vi "zmq REP manual events.vi"() -> ()   [LabVIEW 2018]
uses:
  <vilib>/addons/zeromq/socket_type.ctl
  CAEN_SY527/subvis/Event Sources.ctl
  <vilib>/addons/zeromq/poll_type.ctl
  <vilib>/addons/zeromq/zmq_poll_scalar.vi
  <vilib>/addons/zeromq/zeromq.lvlib
  <vilib>/addons/zeromq/zmq_context.lvclass
  <vilib>/addons/zeromq/zmq_socket.lvclass
panel:
  in  "Send self":bool
  in  "KILL":bool
  in  "Send":bool
  out "h":bool
  out "data":string
  out "error out":errorcluster
  in  "Stop":bool
  in  "ZMQ endpoint":string="tcp://*:5555"
  # "*:5555"
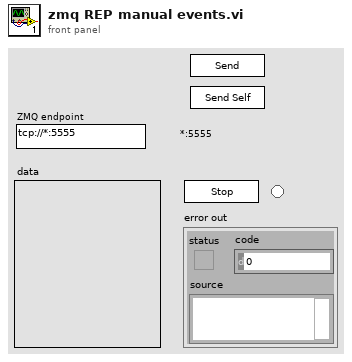
[diagram p1: front panel]
types:
  T1 = typedef "Event Sources.ctl" = enum16{"ZMQ", "INTERNAL", "Check_Errors", "Send_ZMQ_Reply", "Save_PMT_Voltages", "Set_Ramp_Voltage", "Restore PMT Voltages"}
  T2 = typedef "zeromq.lvlib/socket_type.ctl" = enum8{"ZMQ_PAIR", "ZMQ_PUB", "ZMQ_SUB", "ZMQ_REQ", "ZMQ_REP", "ZMQ_DEALER", "ZMQ_ROUTER", "ZMQ_PULL", "ZMQ_PUSH", "ZMQ_XPUB", "ZMQ_XSUB"}
  T3 = typedef "zeromq.lvlib/poll_type.ctl" = enum16{"None", "In", "Out", "In/Out"}
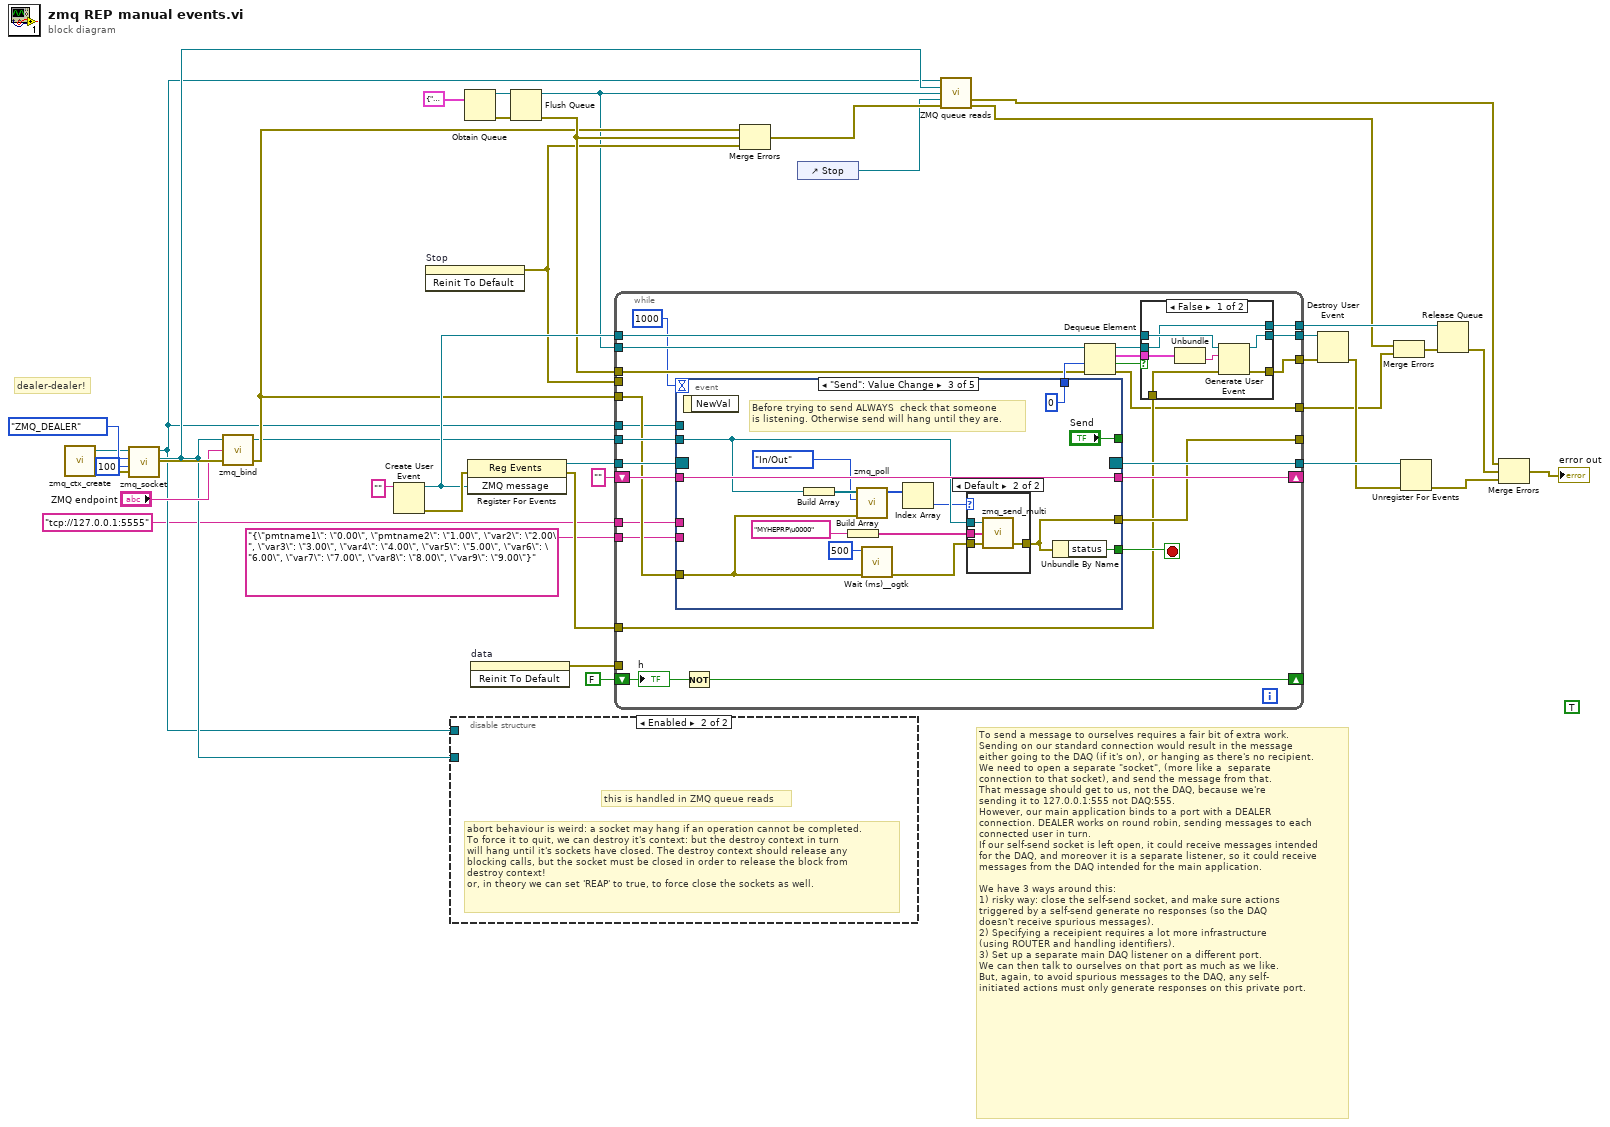
[diagram p0: block diagram]
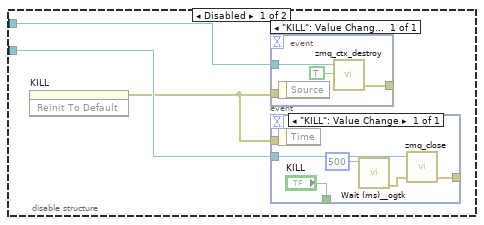
[diagram p2: hidden frame]
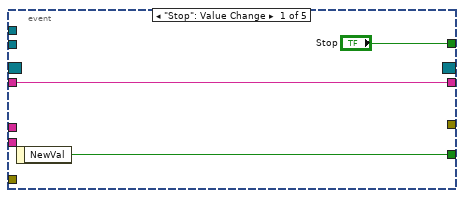
[diagram p4: hidden frame]
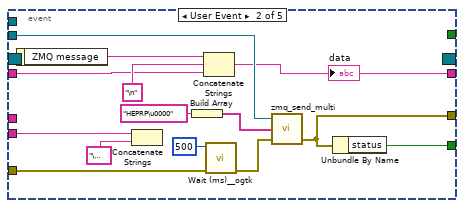
[diagram p5: hidden frame]
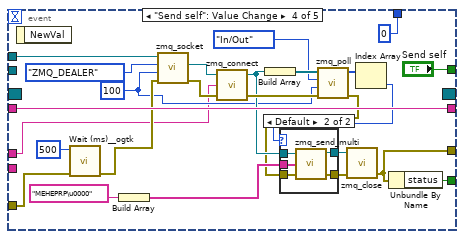
[diagram p7: hidden frame]
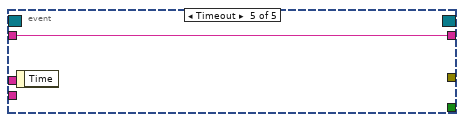
[diagram p9: hidden frame]
diagram:
  (unwired) TRUE
  # "To send a message to ourselves requires a fair bit of extra work.\nSending on our standard connection would result in the message\neither going to the DAQ (if it's on), or hanging as there's no recipient.\nWe need to open a separate \"socket\", (more like a  separate \nconnection to that socket), and send the message from that. \nThat message should get to us, not the DAQ, because we're\nsending it to 127.0.0.1:555 not DAQ:555. \nHowever, our main application binds to a port with a DEALER \nconnection. DEALER works on round robin, sending messages to each\nconnected user in turn. \nIf our self-send socket is left open, it could receive messages intended\nfor the DAQ, and moreover it is a separate listener, so it could receive \nmessages from the DAQ intended for the main application. \n\nWe have 3 ways around this:\n1) risky way: close the self-send socket, and make sure actions\ntriggered by a self-send generate no responses (so the DAQ\ndoesn't receive spurious messages). \n2) Specifying a receipient requires a lot more infrastructure \n(using ROUTER and handling identifiers). \n3) Set up a separate main DAQ listener on a different port.\nWe can then talk to ourselves on that port as much as we like.\nBut, again, to avoid spurious messages to the DAQ, any self-\ninitiated actions must only generate responses on this private port."
  # "dealer-dealer!"
  n1 = call <vilib>:"zmq_ctx_create.vi"() -> ("error out"=w40:errorcluster, "context out"=w35:refnum<class "zmq_context.lvclass">)  [unwired: 4 in]
  n2 = call <vilib>:"zmq_socket.vi"("error in"=w40, "linger (ms)"=100, "socket type"=socket_type."ZMQ_DEALER", "context in"=w35) -> ("error out"=w38:errorcluster, "socket out"=w3:refnum<class "zmq_socket.lvclass">, "context out"=w2:refnum<class "zmq_context.lvclass">)  [unwired: 1 in]
  n3 = call <vilib>:"zmq_bind.vi"("error in"=w38, "endpoint"="ZMQ endpoint", "socket in"=w3) -> ("error out"=w13:errorcluster, "socket out"=w4:refnum<class "zmq_socket.lvclass">)  [unwired: 1 in]
  n4 = Create User Event(user event datatype="" ("ZMQ message")) -> (user event=w25:refnum<user-event>, error out=w36:errorcluster)  [unwired: 1 in]
  n5 = invoke on="Stop" class="Bool (strict)" method="Reinit To Default"() -> (error out=w12:errorcluster)  [unwired: 3 in, 2 out]
  n6 = disable-structure shown="Enabled" {
    disable-tunnel: w2 -> [w43 _]
    disable-tunnel: w3 -> [w42 _]
    frame Disabled {
      n7 = invoke on="KILL" class="Bool" method="Reinit To Default"() -> (error out=w41:errorcluster)  [unwired: 3 in, 2 out]
      n8 = event shown="[0] \"KILL\": Value Change" {
        selector: _ -> [_]
        dyn-events: _ -> [_]
        timeout: _ -> [_]
        tunnel: w43 -> [w51]
        tunnel: w41 -> [_]
        tunnel: [w49] -> _
        event "KILL": Value Change {
          n9 = event-data() -> ()  [unwired: 1 in, 1 out]
          n10 = call <vilib>:"zmq_ctx_destroy.vi"("reap? (F)"=TRUE, "context in"=w51) -> ("error out"=w49:errorcluster)  [unwired: 3 in]
        }
      }
      n11 = event shown="[0] \"KILL\": Value Change" {
        selector: _ -> [_]
        dyn-events: _ -> [_]
        timeout: _ -> [_]
        tunnel: w42 -> [w48]
        tunnel: w41 -> [_]
        tunnel: ["KILL"] -> _
        tunnel: [w46] -> _
        event "KILL": Value Change {
          n12 = event-data() -> ()  [unwired: 1 in, 1 out]
          n13 = call <userlib>:"Wait (ms)__ogtk.vi"("milliseconds to wait"=u32 500) -> ("error out"=w44:errorcluster)  [unwired: 9 in, 1 out]
          n14 = call <vilib>:"zmq_close.vi"("error in"=w44, "socket"=w48) -> ("error out"=w46:errorcluster)  [unwired: 3 in]
        }
      }
    }
    frame Enabled {
      # "abort behaviour is weird: a socket may hang if an operation cannot be completed.\nTo force it to quit, we can destroy it's context: but the destroy context in turn\nwill hang until it's sockets have closed. The destroy context should release any\nblocking calls, but the socket must be closed in order to release the block from\ndestroy context! \nor, in theory we can set 'REAP' to true, to force close the sockets as well."
      # "this is handled in ZMQ queue reads"
    }
  }
  n15 = Obtain Queue(element data type=cluster{"Source":T1, "Command":string} {"Source"=enum."ZMQ", "Command"=""} ("element")) -> (queue out=w7:refnum<queue>, error out=w8:errorcluster)  [unwired: 4 in, 1 out]
  n16 = register-events(error in=w36, w25) -> (reference out=w37:refnum<event-registration>, error out=w20:errorcluster)  [unwired: 1 in]
  n17 = invoke on="data" class="Str" method="Reinit To Default"() -> (error out=w30:errorcluster)  [unwired: 3 in, 2 out]
  n18 = Flush Queue(queue=w7, error in (no error)=w8) -> (queue out=w10:refnum<queue>, error out=w14:errorcluster)  [unwired: 1 out]
  n19 = while {
    tunnel: w37 -> [w76]
    tunnel: w4 -> [w75]
    shift-right: [w73] -> _
    shift-left: "" -> [w72]
    tunnel: [w74] -> w34
    tunnel: w30 -> [_]
    shift-right: [w70] -> _
    shift-left: FALSE ("Stop") -> [w71]
    tunnel: w10 -> [w69]
    tunnel: w25 -> [w66]
    tunnel: [w65] -> w24
    tunnel: [w63] -> w23
    tunnel: [w57] -> w22
    tunnel: w20 -> [w58]
    tunnel: w14 -> [w61]
    tunnel: [w60] -> _
    tunnel: w13 -> [w59]
    tunnel: [w56] -> w16
    tunnel: w12 -> [_]
    tunnel: "{\"pmtname1\": \"0.00\", \"pmtname2\": \"1.00\", \"var2\": \"2.00\", \"var3\": \"3.00\", \"var4\": \"4.00\", \"var5\": \"5.00\", \"var6\": \"6.00\", \"var7\": \"7.00\", \"var8\": \"8.00\", \"var9\": \"9.00\"}" ("JSON string 2") -> [w54]
    tunnel: w2 -> [w53]
    tunnel: "tcp://127.0.0.1:5555" ("String") -> [w52]
    stop <- w77 stop-if-true
    n20 = event shown="[2] \"Send\": Value Change" {
      selector: w76 -> [_ _ _ _ _]
      dyn-events: [_ _ _ _ _] -> w74
      timeout: 1000 -> [_ _ _ _ _]
      tunnel: [w90 w103 w119 w149 _] -> w77
      tunnel: w75 -> [_ w104 w106 _ _]
      tunnel: [w89 w101 w112 w140 w157] -> w73
      tunnel: w72 -> [w89 w100 w112 w140 w157]
      tunnel: [_ w98 w118 w130 _] -> w60
      tunnel: [_ _ 0 ("timeout in ms (-1)") 0 ("timeout in ms (-1)") _] -> w62
      tunnel: w59 -> [_ w96 w107 w147 _]
      tunnel: w54 -> [_ w94 _ _ _]
      tunnel: ["Stop" _ "Send" "Send self" _] -> _
      tunnel: w53 -> [_ _ _ w142 _]
      tunnel: w52 -> [_ _ _ w125 _]
      event "Stop": Value Change {
        n21 = event-data() -> ("NewVal"=w90:bool)  [unwired: 1 in]
      }
      event User Event {
        n22 = event-data() -> ("ZMQ message"=w99:string)  [unwired: 1 in]
        n23 = Concatenate Strings(w94, "\u0000" ("String")) -> ()  [unwired: 1 out]
        n24 = Build Array("HEPRP\u0000" ("String")) -> (w92:string[])
        n25 = Concatenate Strings(w99, "\n" ("String"), w100) -> (w101:string)
        "data" <- w101
        n26 = call <userlib>:"Wait (ms)__ogtk.vi"("error in (no error)"=w96, "milliseconds to wait"=u32 500) -> ("error out"=w97:errorcluster)  [unwired: 8 in, 1 out]
        n27 = call <vilib>:"zmq_send_multi.vi"("error in"=w97, "parts"=w92, "socket in"=w104) -> ("error out"=w98:errorcluster)  [unwired: 1 in, 1 out]
        n28 = Unbundle By Name(w98) -> ("status"=w103:bool)
      }
      event "Send": Value Change {
        # "Before trying to send ALWAYS  check that someone\nis listening. Otherwise send will hang until they are."
        n29 = event-data() -> ()  [unwired: 1 in, 1 out]
        n30 = Build Array(w106) -> (w110:refnum<class "zmq_socket.lvclass">[])
        n31 = Build Array("MYHEPRP\u0000" ("String")) -> (w114:string[])
        n32 = call-poly <vilib>:"zmq_poll.vi"("error in"=w107, "poll type"=poll_type."In/Out", "sockets"=w110) -> ("polled events"=w109:T3[])  [unwired: 1 in, 3 out]
        n33 = call <userlib>:"Wait (ms)__ogtk.vi"("error in (no error)"=w107, "milliseconds to wait"=u32 500) -> ("error out"=w117:errorcluster)  [unwired: 8 in, 1 out]
        n34 = Index Array(array=w109) -> (element=w105:T3)  [unwired: 1 in]
        n35 = case shown="Default" w105 {
          tunnel: [w120 w124] -> w118
          tunnel: w117 -> [w120 w123]
          tunnel: w114 -> [_ w122]
          tunnel: w106 -> [_ w121]
          frame "None" {
          }
          frame Default {
            n36 = call <vilib>:"zmq_send_multi.vi"("error in"=w123, "parts"=w122, "socket in"=w121) -> ("error out"=w124:errorcluster)  [unwired: 1 in, 1 out]
          }
        }
        n37 = Unbundle By Name(w118) -> ("status"=w119:bool)
      }
      event "Send self": Value Change {
        w126 = 100 ("linger (ms)")
        n38 = event-data() -> ()  [unwired: 1 in, 1 out]
        n39 = call <userlib>:"Wait (ms)__ogtk.vi"("error in (no error)"=w147, "milliseconds to wait"=u32 500) -> ("error out"=w134:errorcluster)  [unwired: 8 in, 1 out]
        n40 = Build Array("MEHEPRP\u0000" ("String")) -> (w145:string[])
        n41 = call <vilib>:"zmq_socket.vi"("error in"=w134, "linger (ms)"=w126, "socket type"=socket_type."ZMQ_DEALER", "context in"=w142) -> ("error out"=w135:errorcluster, "socket out"=w139:refnum<class "zmq_socket.lvclass">)  [unwired: 1 in, 1 out]
        n42 = call <vilib>:"zmq_connect.vi"("error in"=w135, "endpoint"=w125, "socket in"=w139) -> ("error out"=w138:errorcluster, "socket out"=w136:refnum<class "zmq_socket.lvclass">)  [unwired: 1 in]
        n43 = Build Array(w136) -> (w137:refnum<class "zmq_socket.lvclass">[])
        n44 = call-poly <vilib>:"zmq_poll.vi"("error in"=w138, "timeout"=w126, "poll type"=poll_type."In/Out", "sockets"=w137) -> ("error out"=w133:errorcluster, "polled events"=w132:T3[])  [unwired: 2 out]
        n45 = Index Array(array=w132) -> (element=w131:T3)  [unwired: 1 in]
        n46 = case shown="Default" w131 {
          tunnel: [w151 w156] -> w129
          tunnel: w145 -> [_ w155]
          tunnel: w136 -> [w150 w154]
          tunnel: w133 -> [w151 w153]
          tunnel: [w150 w152] -> w128
          frame "None" {
          }
          frame Default {
            n47 = call <vilib>:"zmq_send_multi.vi"("error in"=w153, "parts"=w155, "socket in"=w154) -> ("error out"=w156:errorcluster, "socket out"=w152:refnum<class "zmq_socket.lvclass">)  [unwired: 1 in]
          }
        }
        n48 = call <vilib>:"zmq_close.vi"("error in"=w129, "socket"=w128) -> ("error out"=w130:errorcluster)  [unwired: 3 in]
        n49 = Unbundle By Name(w130) -> ("status"=w149:bool)
      }
      event Timeout {
        n50 = event-data() -> ()  [unwired: 1 in, 1 out]
      }
    }
    n51 = Not(x=w71) -> (.not. x?=w70:bool)
    n52 = Dequeue Element(queue=w69, timeout in ms (-1)=w62, error in (no error)=w61) -> (queue out=w64:refnum<queue>, element=w67:cluster{"Source":T1, "Command":string}, timed out?=w68:bool, error out=w56:errorcluster)
    n53 = case shown="False" w68 {
      tunnel: w67 -> [w79 _]
      tunnel: w66 -> [w84 w87]
      tunnel: [w83 w85] -> w57
      tunnel: [w82 w87] -> w65
      tunnel: w64 -> [w81 w86]
      tunnel: [w81 w86] -> w63
      tunnel: w58 -> [w80 w85]
      frame False {
        n54 = Unbundle(w79) -> ("Command"=w78:string)  [unwired: 1 out]
        n55 = Generate User Event(user event=w84, event data cluster=w78, error in=w80) -> (user event out=w82:refnum<user-event>, error out=w83:errorcluster)  [unwired: 1 in]
      }
      frame True {
      }
    }
    "h" <- w71
  }
  n56 = Merge Errors(w13, w14, w12) -> (w11:errorcluster)
  n57 = control-ref of="Stop"() -> (w9:refnum<vi>)
  n58 = call "ZMQ queue reads.vi"("context in"=w2, "zmq_socket in"=w3, "queue in"=w10, "Stop"=w9, "Error in"=w11) -> ("ZMQ error out"=w5:errorcluster, "Queue error out"=w17:errorcluster)  [unwired: 8 in, 1 out]
  n59 = Destroy User Event(user event=w24, error in=w22) -> (error out=w19:errorcluster)
  n60 = Merge Errors(w17, w16) -> (w18:errorcluster)
  n61 = Unregister For Events(event registration refnum=w34, error in=w19) -> (error out=w32:errorcluster)
  n62 = Release Queue(queue=w23, error in (no error)=w18) -> (error out=w21:errorcluster)  [unwired: 1 in, 2 out]
  n63 = Merge Errors(w5, w21, w32) -> (→"error out":errorcluster)
